vi "RoomBeaconToIndex.vi"(8 "error in (no error)":errorcluster, 10 "Beacon Id":string, 11 "Rooms In":refnum<class "Room.lvclass">[](array[class])) -> (0 "error out":errorcluster, 2 "Index":i32, 3 "Rooms Out":refnum<class "Room.lvclass">[](array[class]))   [LabVIEW 2015]
uses:
  Room.lvclass
  Room.lvclass/Room.ctl
  Read Beacon Id.vi
  <vilib>/Utility/error.llb/Error Cluster From Error Code.vi
  <vilib>/ErrorRing/Error Ring.xnode
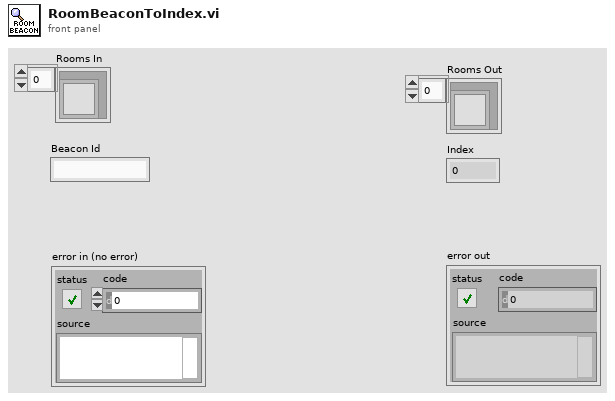
[diagram p1: front panel]
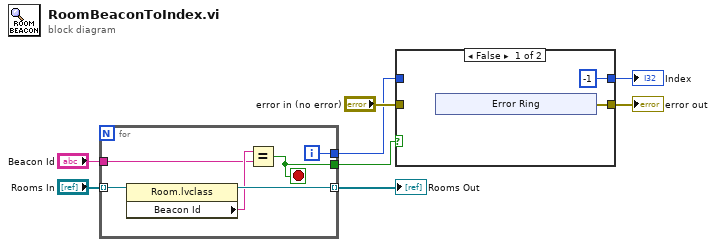
[diagram p0: block diagram]
diagram:
  n1 = for {
    tunnel: [w13] -> w8 mode=indexing
    tunnel: "Rooms In" -> [w14] mode=indexing
    tunnel: [w11] -> w3
    tunnel: [w10] -> w1
    tunnel: "Beacon Id" -> [w9]
    i -> [w10]
    stop <- w11 stop-if-true
    n2 = property class="Room.lvclass"(reference=w14) -> (reference out=w13:refnum<class "Room.lvclass">, "Beacon Id"=w12:string)  [unwired: 1 in, 1 out]
    n3 = Equal?(x=w12, y=w9) -> (x = y?=w11:bool)
  }
  "Rooms Out" <- w8
  n4 = case shown="False" w3 {
    tunnel: "error in (no error)" -> [_ w23]
    tunnel: [w16 w23] -> w4
    tunnel: [-1 ("f") w22] -> w2
    tunnel: w1 -> [_ w22]
    frame False {
      n5 = xnode "Error Ring"() -> ("error out"=w16:errorcluster)
    }
    frame True {
    }
  }
  "Index" <- w2
  "error out" <- w4
